vi "Test Plugin Parameter Default Value Persisted.vi"(8 "error in (no error)":errorcluster, 11 "Configuration Manager Test in":refnum<class "Configuration Manager Test.lvclass">) -> (0 "error out":errorcluster, 3 "Configuration Manager Test out":refnum<class "Configuration Manager Test.lvclass">)   [LabVIEW 2020, in "Configuration Manager Test.lvclass"]
uses:
  Configuration Manager Test.lvclass
  Configuration Manager Test.lvclass/Configuration Manager Test.ctl
  source/User Interface/Configuration Manager/Configuration Manager.lvclass
  da4b3e93-04f0-485b-8eef-eaf6a6b0a3f6.vi
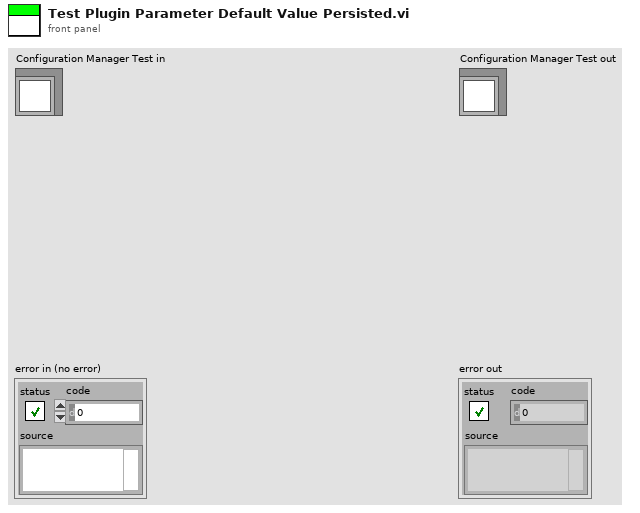
[diagram p1: front panel]
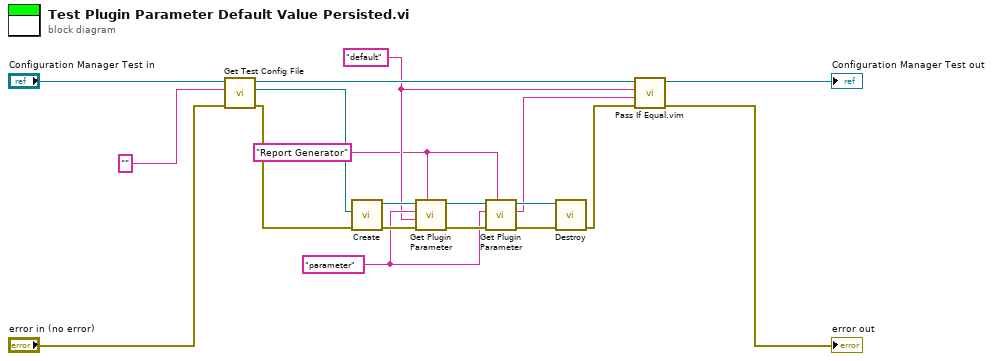
[diagram p0: block diagram]
diagram:
  w1 = "Report Generator"
  w3 = "default" ("Default Value")
  w5 = "parameter" ("Name")
  n1 = call "Get Test Config File.vi"("error in (no error)"="error in (no error)", "File Content"="", "Configuration Manager Test in"="Configuration Manager Test in") -> ("error out"=w14:errorcluster, "File Path"=w9:path, "Configuration Manager Test out"=w11:refnum<class "Configuration Manager Test.lvclass">)  [unwired: 6 in]
  n2 = call "Create.vi"("error in (no error)"=w14, "configuration file path"=w9) -> ("error out"=w16:errorcluster, "Configuration Manager out"=w17:refnum<class "Configuration Manager.lvclass">)  [unwired: 8 in]
  n3 = call "Get Plugin Parameter.vi"("Plugin"=w1, "error in (no error)"=w16, "Default Value"=w3, "Name"=w5, "Configuration Manager in"=w17) -> ("error out"=w15:errorcluster, "Configuration Manager out"=w7:refnum<class "Configuration Manager.lvclass">)  [unwired: 4 in, 1 out]
  n4 = call "Get Plugin Parameter.vi"("Plugin"=w1, "error in (no error)"=w15, "Name"=w5, "Configuration Manager in"=w7) -> ("error out"=w8:errorcluster, "Value"=w4:string, "Configuration Manager out"=w6:refnum<class "Configuration Manager.lvclass">)  [unwired: 5 in]
  n5 = call "Destroy.vi"("error in (no error)"=w8, "Configuration Manager In"=w6) -> ("error out"=w13:errorcluster)  [unwired: 9 in]
  n6 = call "Pass If Equal.vim"("error in (no error)"=w13, "Actual"=w4, "Expected"=w3, "LUnit Test Case In"=w11) -> ("error out"=→"error out":errorcluster, "LUnit Test Case Out"=→"Configuration Manager Test out":refnum<class "Configuration Manager Test.lvclass">)  [unwired: 6 in]
